vi "04. Native MQTT Streaming Client.vi"() -> ()   [LabVIEW 2019]
uses:
  streaming-request -- cluster.ctl
  Actor/Response -- cluster.ctl
  <vilib>/LabVIEW Open Source Project/MQTT Control Packets/Control Packets/ControlPacket/ControlPacket.lvclass/ControlPacket.ctl
  2ad39a46-4504-4743-a052-40662866620d.vi
  eb8eb180-2280-4b70-97f6-c873bf82b039.vi
  6c5966a4-9c55-4462-a978-28a450dbad44.vi
  <vilib>/LabVIEW Open Source Project/MQTT Control Packets/Control Packets/PUBLISH/PUBLISH.lvclass
  C:/Program Files (x86)/National Instruments/LabVIEW 2019/vi.lib/LabVIEW Open Source Project/MQTT Control Packets/Control Packets/ControlPacket/ControlPacket.lvclass
  <vilib>/JDP Science/JSONtext/Variant to JSON Text.vi
  <vilib>/JDP Science/JSONtext/JSON text to Variant.vi
  <vilib>/JDP Science/JSONtext/LVClass Serializer/JSONtext LVClass Serializer.lvclass
  <vilib>/LabVIEW Open Source Project/MQTT Control Packets/Control Packets/ControlPacket/ControlPacket.lvclass
  <vilib>/LabVIEW Open Source Project/Unicity/RandomStringGenerator/RandomStringGenerator.lvclass
panel:
  in  "Clear":bool
  in  "History":i32(listbox)
  in  "Streaming Service Namespace":string="demo/stream"
  out "Topic":string
  in  "filename":string="filename.tdms"
  in  "Download":bool
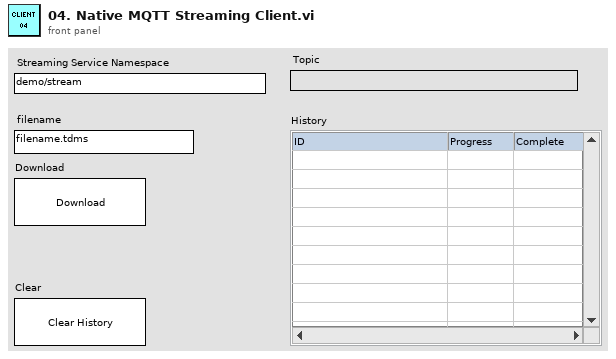
[diagram p1: front panel]
types:
  T1 = map{string, cluster{"progress (%)":dbl, "complete":bool, "error":bool}}
  T2 = typedef "Actor Private Data.ctl" = cluster{"Client":refnum<class "Client.lvclass">, "QualifiedName":string, "EventReg":refnum<event-registration>, "Private Events":T3}
  T3 = typedef "Actor Private Events -- cluster.ctl" = cluster{"Stop":refnum<user-event>, "Subscribe":refnum<user-event>, "Unsubscribe":refnum<user-event>, "publish":refnum<user-event>}
  T4 = typedef "streaming-request -- cluster.ctl" = cluster{"uri":string, "filepath":string, "update-topic":string, "id":string}
  T5 = cluster{"progress (%)":dbl, "complete":bool, "error":bool}
  T6 = typedef "Response -- cluster.ctl" = cluster{"<JSON>result":string, "id":string, "<JSON>error":string}
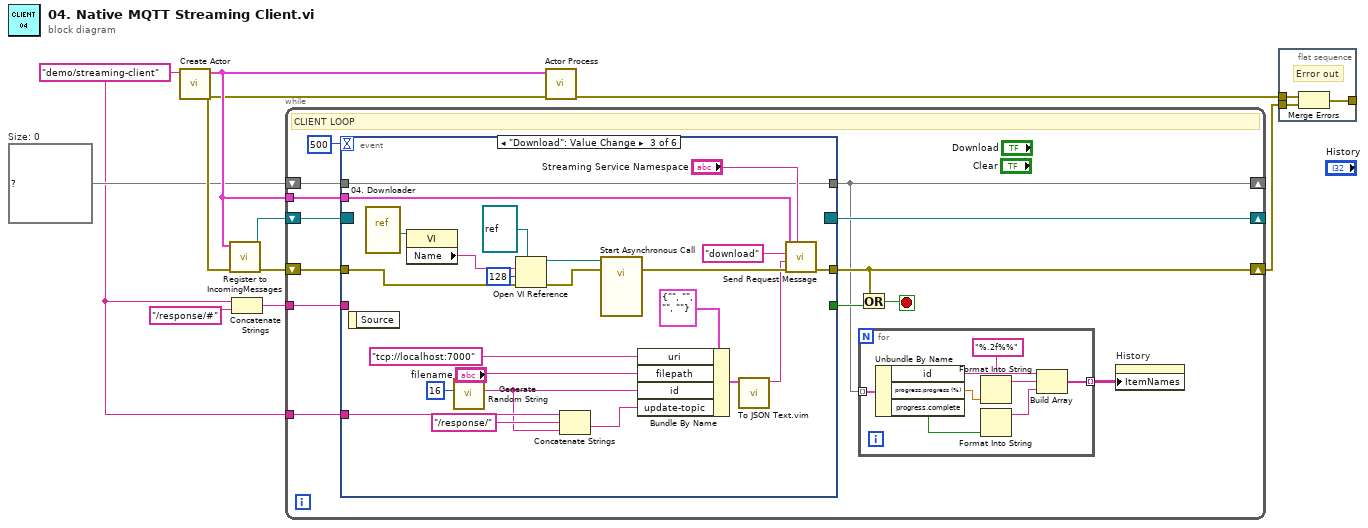
[diagram p0: block diagram]
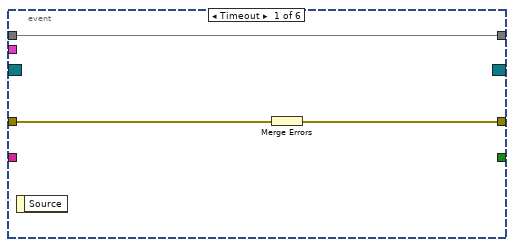
[diagram p2: hidden frame]
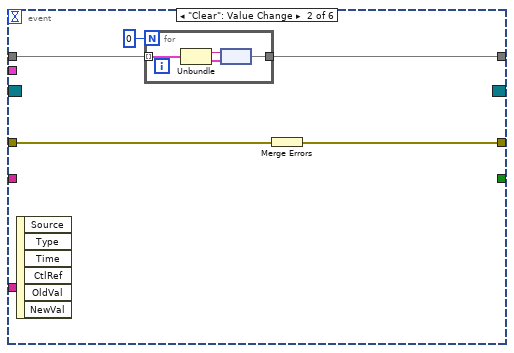
[diagram p3: hidden frame]
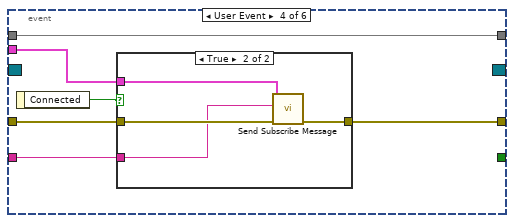
[diagram p4: hidden frame]
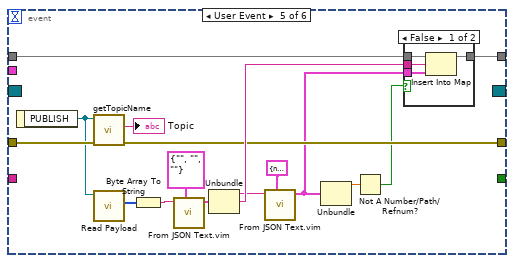
[diagram p6: hidden frame]
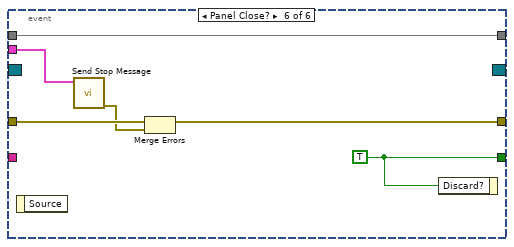
[diagram p8: hidden frame]
diagram:
  w2 = T1 {}  # Size: 0
  w1 = "demo/streaming-client" ("QualifiedName")
  n1 = call "Create Actor.vi"("QualifiedName"=w1) -> ("error out"=w5:errorcluster, "Actor Class"=w9:T2)  [unwired: 9 in]
  n2 = call "Register to IncomingMessages.vi"("error in"=w5, "Actor Class"=w9) -> ("error out"=w8:errorcluster, "Incoming Messages"=w10:refnum<event-registration>)  [unwired: 8 in]
  n3 = Concatenate Strings(w1, "/response/#" ("QualifiedName")) -> (w3:string)
  n4 = while {
    tunnel: w9 -> [w21]
    shift-right: [w18] -> _
    shift-left: w10 -> [w19]
    shift-right: [w16] -> w7
    shift-left: w8 -> [w17]
    tunnel: w3 -> [w15]
    shift-right: [w12] -> _
    shift-left: w2 -> [w14]
    tunnel: w1 -> [w13]
    stop <- w22 stop-if-true
    # "CLIENT LOOP"
    n5 = event shown="[2] \"Download\": Value Change" {
      selector: w19 -> [_ _ _ _ _ _]
      dyn-events: [_ _ _ _ _ _] -> w18
      timeout: 500 -> [_ _ _ _ _ _]
      tunnel: [_ _ _ _ _ w104] -> w23
      tunnel: w21 -> [_ _ w65 w70 _ w103]
      tunnel: [w33 w38 w66 w71 w82 w100] -> w16
      tunnel: w17 -> [w34 w39 w48 w72 w93 w102]
      tunnel: w15 -> [_ _ _ w68 _ _]
      tunnel: w14 -> [w32 w35 w46 w67 w86 w99]
      tunnel: [w32 w36 w46 w67 w83 w99] -> w12
      tunnel: w13 -> [_ _ w59 _ _ _]
      event Timeout {
        n6 = event-data() -> ()  [unwired: 1 in, 1 out]
        n7 = Merge Errors(w34) -> (w33:errorcluster)
      }
      event "Clear": Value Change {
        n8 = event-data() -> ()  [unwired: 1 in, 6 out]
        n9 = for {
          N: 0 -> [_]
          tunnel: w35 -> [w43] mode=indexing
          tunnel: [w40] -> w36
          n10 = Unbundle(w43) -> ("id"=w42:string, "progress"=w41:T5)
          n11 = node(w42, w41) -> (w40:T1)
        }
        n12 = Merge Errors(w39) -> (w38:errorcluster)
      }
      event "Download": Value Change {
        n13 = event-data() -> ()  [unwired: 1 in, 1 out]
        n14 = vi-ref "04. Downloader.vi"() -> (w54:refnum<vi>)
        n15 = property class="VI"(reference=w54) -> ("Name"=w53:string)  [unwired: 1 in, 2 out]
        n16 = call <vilib>:"Generate Random String.vi"("String Length (32)"=u32 16) -> ("Random String"=w57:string)  [unwired: 10 in]
        n17 = Open VI Reference(type specifier VI Refnum (for type only)=refnum<vi> refnum, vi path=w53, options=128, error in (no error)=w48) -> (vi reference=w51:refnum<vi>, error out=w50:errorcluster)  [unwired: 2 in]
        n18 = Concatenate Strings(w59, "/response/" ("QualifiedName"), w57) -> (w56:string)
        n19 = call-by-ref "Start Asynchronous Call"(reference=w51, error in=w50) -> (error out=w47:errorcluster)  [unwired: 11 in, 2 out]
        n20 = Bundle By Name(cluster=T4 {"uri"="", "filepath"="", "update-topic"="", "id"=""} ("streaming-request"), "uri"="tcp://localhost:7000", "filepath"="filename", "id"=w57, "update-topic"=w56) -> (w45:T4)
        n21 = call "To JSON Text.vim"("Anything"=w45) -> ("<JSON>"=w44:string)  [unwired: 9 in, 1 out]
        n22 = call "Send Request Message.vi"("Qualified Name"="Streaming Service Namespace", "error in"=w47, "<JSON>params"=w44, "method"="download", "Actor Class"=w65) -> ("error out"=w66:errorcluster)  [unwired: 4 in, 2 out]
      }
      event User Event {
        n23 = event-data() -> ("Connected"=w69:bool)  [unwired: 1 in]
        n24 = case shown="True" w69 {
          tunnel: w72 -> [w73 w77]
          tunnel: [w73 w76] -> w71
          tunnel: w70 -> [_ w75]
          tunnel: w68 -> [_ w74]
          frame False {
          }
          frame True {
            n25 = call "Send Subscribe Message.vi"("error in"=w77, "Topic"=w74, "Actor Class"=w75) -> ("error out"=w76:errorcluster)  [unwired: 8 in]
          }
        }
      }
      event User Event {
        n26 = event-data() -> ("PUBLISH"=w92:refnum<class "PUBLISH.lvclass">)  [unwired: 1 in]
        n27 = call <vilib>:"getTopicName.vi"("error in (no error)"=w93, "PUBLISH in"=w92) -> ("error out"=w82:errorcluster, "Topic"=→"Topic":string)  [unwired: 7 in, 1 out]
        n28 = call <vilib>:"Read Payload.vi"("ControlPacket in"=w92) -> ("Payload"=w91:u8[])  [unwired: 9 in, 1 out]
        n29 = Byte Array To String(unsigned byte array=w91) -> (string=w89:string)
        n30 = call "From JSON Text.vim"("Data Type and Default Value"=T6 {"<JSON>result"="", "id"="", "<JSON>error"=""} ("response"), "JSON"=w89) -> ("Data out"=w87:T6)  [unwired: 8 in, 1 out]
        n31 = Unbundle(w87) -> ("<JSON>result"=w84:string, "id"=w85:string)  [unwired: 1 out]
        n32 = call "From JSON Text.vim"("Data Type and Default Value"=T5 {"progress (%)"=nan, "complete"=FALSE, "error"=FALSE}, "JSON"=w84) -> ("Data out"=w80:T5)  [unwired: 8 in, 1 out]
        n33 = Unbundle(w80) -> ("progress (%)"=w79:dbl)  [unwired: 2 out]
        n34 = Not A Number/Path/Refnum?(number/path/refnum=w79) -> (NaN/Path/Refnum?=w78:bool)
        n35 = case shown="False" w78 {
          tunnel: w86 -> [w97 w98]
          tunnel: w85 -> [w96 _]
          tunnel: [w95 w98] -> w83
          tunnel: w80 -> [w94 _]
          frame False {
            n36 = Insert Into Map(map in=w97, key=w96, value=w94) -> (map out=w95:T1)  [unwired: 2 out]
          }
          frame True {
          }
        }
      }
      event Panel Close? {
        w104 = TRUE ("Discard?")
        n37 = event-data() -> ()  [unwired: 1 in, 1 out]
        n38 = call "Send Stop Message.vi"("Actor Class"=w103) -> ("error out"=w101:errorcluster)  [unwired: 10 in]
        n39 = Merge Errors(w102, w101) -> (w100:errorcluster)
        n40 = event-data("Discard?"=w104) -> ()  [unwired: 1 in, 1 out]
      }
    }
    n41 = Or(x=w16, y=w23) -> (x .or. y?=w22:bool)
    n42 = for {
      tunnel: w12 -> [w31] mode=indexing
      tunnel: [w24] -> w11 mode=indexing
      n43 = Unbundle By Name(w31) -> ("id"=w29:string, "progress.progress (%)"=w26:dbl, "progress.complete"=w30:bool)
      n44 = Format Into String(format string="%.2f%%", w26) -> (resulting string=w28:string)  [unwired: 2 in, 1 out]
      n45 = Format Into String(w30) -> (resulting string=w27:string)  [unwired: 3 in, 1 out]
      n46 = Build Array(w29, w28, w27) -> (w24:string[])
    }
    n47 = property on="History" class="MCListbox (strict)"("ItemNames"=w11) -> ()  [unwired: 2 in, 2 out]
  }
  n48 = call "Actor Process.vi"("error in"=w5, "Actor Class"=w9) -> ("error out"=w6:errorcluster)  [unwired: 9 in]
  n49 = flat-sequence {
    tunnel: w6 -> [w107]
    tunnel: w7 -> [w106]
    tunnel: [w105] -> _
    frame #0 {
      # "Error out"
      n50 = Merge Errors(w107, w106) -> (w105:errorcluster)
    }
  }
